vi "Vizulize_exp.vi"(10 "ControlQueue":refnum<queue>, 11 "Message in":refnum<class "Message.lvclass">) -> ()   [LabVIEW 2015]
uses:
  Message/Message.lvclass
  controls/SliderSDII.ctl
  controls/Del.ctl
  controls/Add.ctl
  dependecies/ControlsVIs/Clusters-def/Standard Command.ctl
panel:
  in  "times slider":T1={120.7741935483871, 734.8387096774194} scale=-250.0..4235.0 scale format="%#.1f"
  in  "del spec":i32=2 min=2 step=1
  in  "Del spectrum":T2
  in  "Add spectrum":T3
  out "Spectra":cluster{"Y":dbl[], "Y":dbl[]}[](graph)
  in  "waves slider":T1={434.19354838709677, 734.8387096774194} scale=240.82404..813.94461 scale format="%#.1f"
  in  "del kin":i32=2 min=2 step=1
  in  "LogY":bool
  in  "Del kinetics":T2
  in  "Add kinetics":T3
  out "Kinetics":cluster{"Y":dbl[], "Y":dbl[]}[](graph)
  out "Received command":string
  out "Exp data graph":dbl[][](graph)
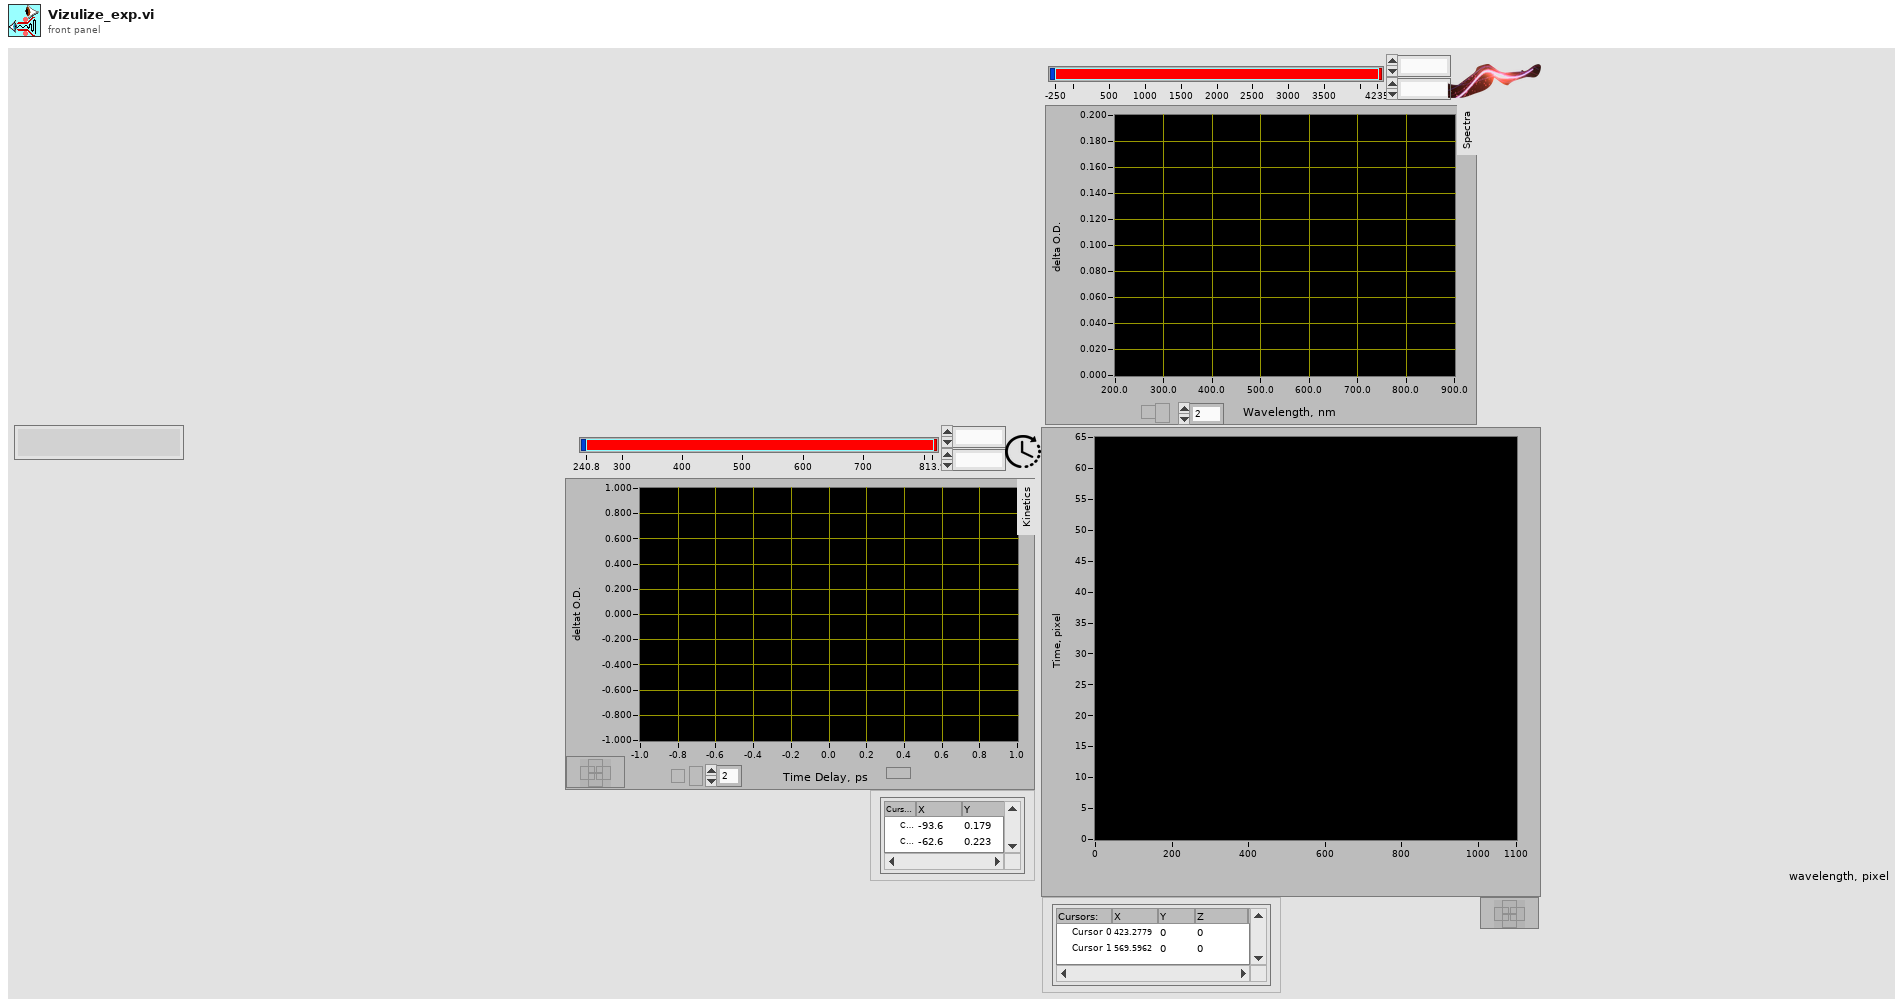
[diagram p1: front panel]
types:
  T1 = typedef "SliderSDII.ctl" = cluster{dbl, dbl}
  T2 = typedef "Del.ctl" = bool
  T3 = typedef "Add.ctl" = bool
  T4 = typedef "Standard Command.ctl" = cluster{"command":string, "data":variant}
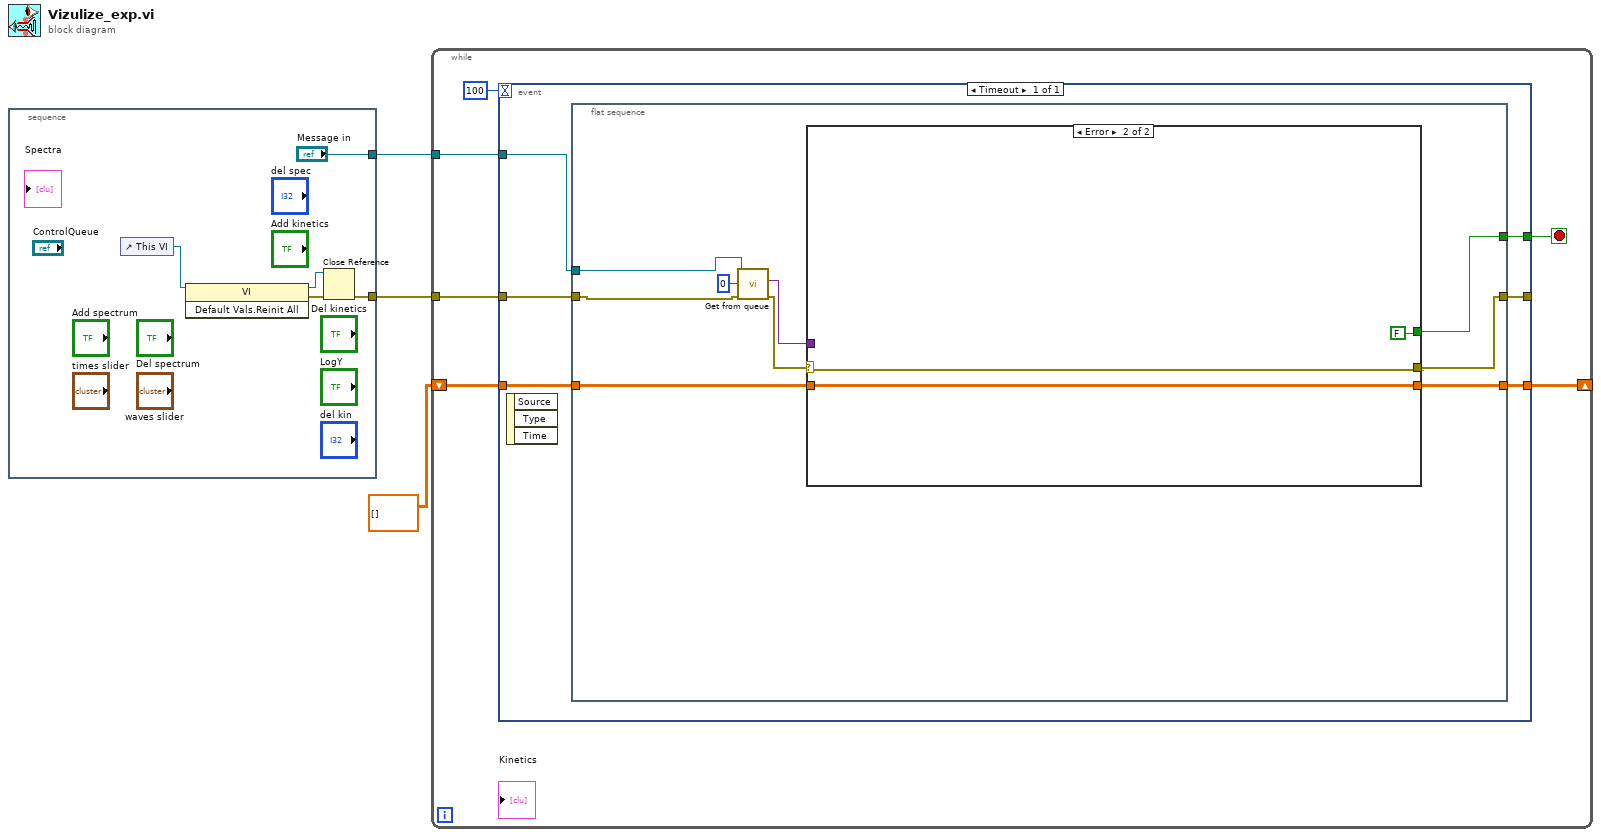
[diagram p0: block diagram]
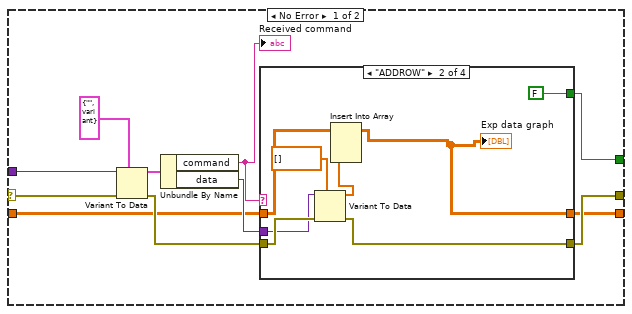
[diagram p2: hidden frame]
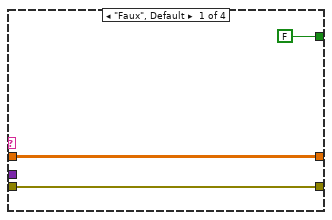
[diagram p3: hidden frame]
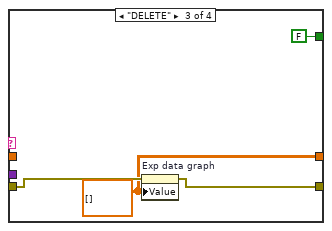
[diagram p4: hidden frame]
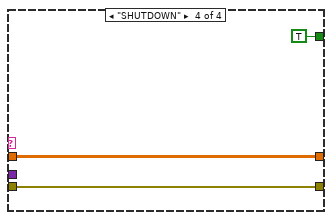
[diagram p5: hidden frame]
diagram:
  n1 = stacked-sequence {
    tunnel: [w5] -> w3
    tunnel: ["Message in"] -> w2
    frame #0 {
      n2 = control-ref of="This VI"() -> (w6:refnum<vi>)
      n3 = invoke class="VI" method="Default Vals.Reinit All"(reference=w6) -> (reference out=w7:refnum<vi>, error out=w8:errorcluster)  [unwired: 2 in, 1 out]
      n4 = Close Reference(reference=w7, error in (no error)=w8) -> (error out=w5:errorcluster)
    }
  }
  n5 = while {
    tunnel: w3 -> [w12]
    tunnel: w2 -> [w11]
    shift-right: [w9] -> _
    shift-left: dbl[][] [] ("Exp data graph") -> [w10]
    stop <- w14 stop-if-true
    n6 = event shown="[0] Timeout" {
      selector: _ -> [_]
      dyn-events: _ -> [_]
      timeout: 100 -> [_]
      tunnel: [w19] -> _
      tunnel: [w20] -> w14
      tunnel: w12 -> [w18]
      tunnel: w11 -> [w17]
      tunnel: w10 -> [w16]
      tunnel: [w15] -> w9
      event Timeout {
        n7 = event-data() -> ()  [unwired: 1 in, 3 out]
        n8 = flat-sequence {
          tunnel: [w26] -> w20
          tunnel: [w25] -> w19
          tunnel: w18 -> [w23]
          tunnel: w17 -> [w24]
          tunnel: w16 -> [w22]
          tunnel: [w21] -> w15
          frame #0 {
            n9 = call "Get from queue.vi"("error in (no error)"=w23, "timeout in ms (-1)"=0, "Message in"=w24) -> ("error out"=w27:errorcluster, "Data"=w28:variant)  [unwired: 6 in, 1 out]
            n10 = case shown="Error" w27 {
              selector: w27 -> [w40 w60]
              tunnel: w28 -> [w35 _]
              tunnel: [w32 w60] -> w25
              tunnel: [w34 FALSE] -> w26
              tunnel: w22 -> [w31 w59]
              tunnel: [w30 w59] -> w21
              frame No Error {
                n11 = Variant To Data(error in=w40, type=T4 {"command"="", "data"=variant} ("input cluster"), Variant=w35) -> (data=w38:T4, error out=w36:errorcluster)
                n12 = Unbundle By Name(w38) -> ("command"=w33:string, "data"=w37:variant)
                "Received command" <- w33
                n13 = case shown="\"ADDROW\"" w33 {
                  tunnel: [w43 w49 w54 w57] -> w32
                  tunnel: [FALSE FALSE FALSE TRUE] -> w34
                  tunnel: w37 -> [_ w45 _ _]
                  tunnel: w36 -> [w43 w50 w55 w57]
                  tunnel: w31 -> [w41 w48 _ w56]
                  tunnel: [w41 w44 w52 w56] -> w30
                  frame "Faux", Default {
                  }
                  frame "ADDROW" {
                    n14 = Variant To Data(error in=w50, type=dbl[] [] ("new element/subarray"), Variant=w45) -> (data=w46:dbl[], error out=w49:errorcluster)
                    n15 = Insert Into Array(array=w48, new element=w46) -> (w44:dbl[][])  [unwired: 2 in]
                    "Exp data graph" <- w44
                  }
                  frame "DELETE" {
                    w52 = dbl[][] [] ("Exp data graph")
                    n16 = property on="Exp data graph" class="IntGraph (strict)"(error in=w55, "Value"=w52) -> (error out=w54:errorcluster)  [unwired: 1 in, 1 out]
                  }
                  frame "SHUTDOWN" {
                  }
                }
              }
              frame Error {
              }
            }
          }
        }
      }
    }
  }
